vi "Set Top Level Path.vi"(8 "error in (no error)":errorcluster, 10 "Top Level Path":path, 11 "Abstract Model in":refnum<class "Abstract Model.lvclass">) -> (0 "error out":errorcluster, 3 "Abstract Model out":refnum<class "Abstract Model.lvclass">)   [LabVIEW 2013, in "Abstract Model.lvlib" / "Abstract Model.lvclass"]
uses:
  Abstract Model.lvclass
  Abstract Model.lvclass/Abstract Model.ctl
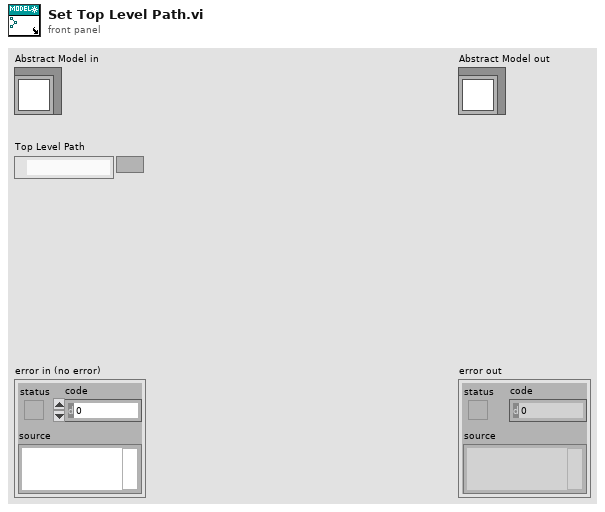
[diagram p1: front panel]
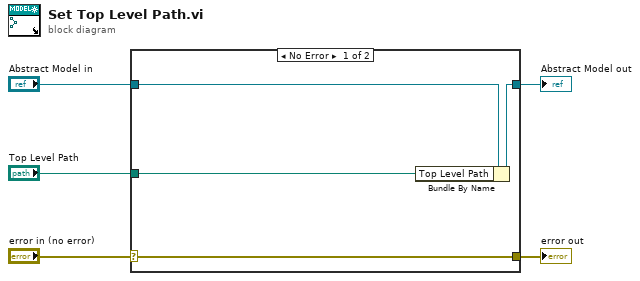
[diagram p0: block diagram]
diagram:
  n1 = case shown="No Error" "error in (no error)" {
    selector: "error in (no error)" -> [w9 w10]
    tunnel: [w9 w10] -> w4
    tunnel: [w7 w11] -> w2
    tunnel: "Abstract Model in" -> [w8 w11]
    tunnel: "Top Level Path" -> [w6 _]
    frame No Error {
      n2 = Bundle By Name(cluster=w8, "Top Level Path"=w6) -> (w7:refnum<class "Abstract Model.lvclass">)
    }
    frame Error {
    }
  }
  "error out" <- w4
  "Abstract Model out" <- w2
